vi "UDP Data Link - RTMs - Remove Channels.vi"(8 "error in (no error)":errorcluster, 11 "Node Ptr":u64 format="%.0x") -> (0 "error out":errorcluster)   [LabVIEW 2012, in "UDP Data Link System Explorer.lvlib"]
uses:
  UDP Data Link System Explorer.lvlib
  <vilib>/NI Veristand/Custom Device API/Get Item Property (I32 Array).vi
  <vilib>/NI Veristand/Custom Device API/Get Item Property (String Array).vi
  <vilib>/NI Veristand/Custom Device API/Set Item Property (I32 Array).vi
  Shared/UDP Data Link Global.vi
  <vilib>/NI Veristand/Custom Device API/Custom Device API.lvlib
  Shared/UDP Data Link Shared.lvlib
  <vilib>/NI Veristand/Custom Device Tools/Custom Device Utility Library/Custom Device Utility Library.lvlib
panel:
  in  "Tag":string
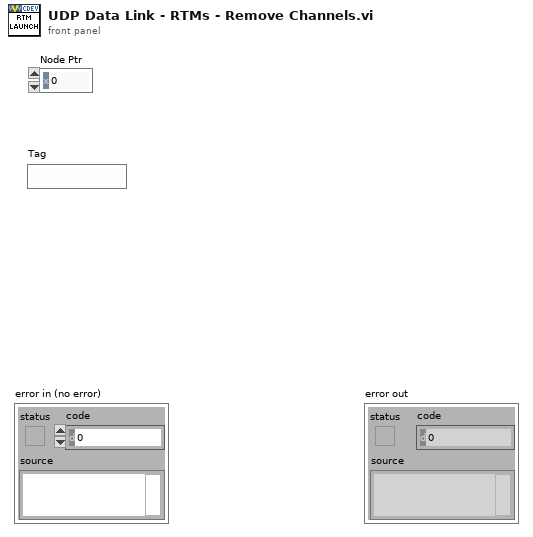
[diagram p1: front panel]
types:
  T1 = typedef "Custom Device API.lvlib/Custom Device Item Ref.ctl" = u64
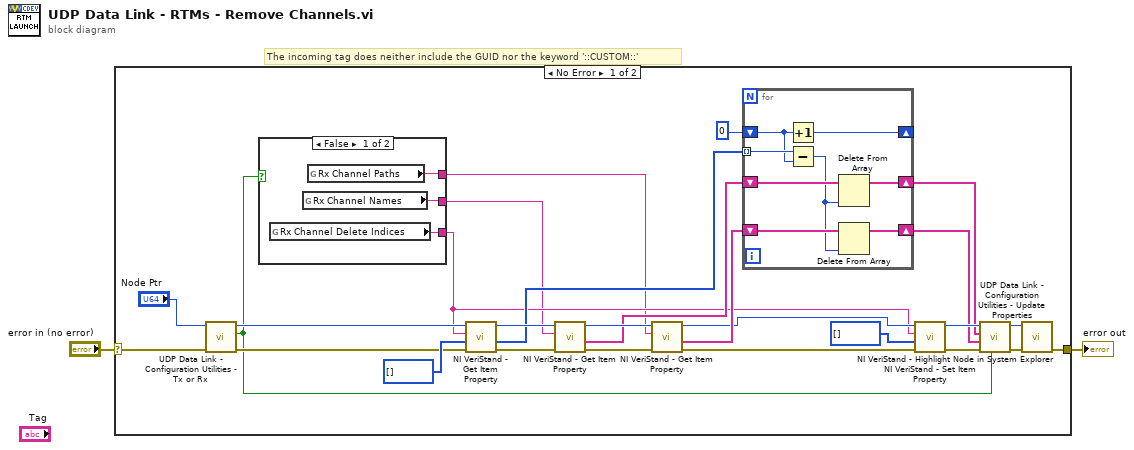
[diagram p0: block diagram]
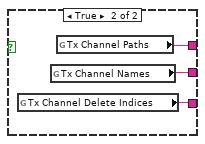
[diagram p2: hidden frame]
diagram:
  # "The incoming tag does neither include the GUID nor the keyword '::CUSTOM::'"
  n1 = case shown="No Error" "error in (no error)" {
    selector: "error in (no error)" -> [w10 w44]
    tunnel: [w18 w44] -> w2
    frame No Error {
      n2 = call "UDP Data Link - Configuration Utilities - Tx or Rx.vi"("error in (no error)"=w10, "Item Ref in"="Node Ptr") -> ("error out"=w7:errorcluster, "Tx?"=w3:bool, "Item Ref out"=w8:T1)  [unwired: 7 in]
      n3 = case shown="False" w3 {
        tunnel: [w32 w35] -> w6
        tunnel: [w31 w34] -> w5
        tunnel: [w30 w33] -> w4
        frame False {
          n4 = global read "UDP Data Link Global.vi" "Rx Channel Delete Indices"() -> (w32:string)
          n5 = global read "UDP Data Link Global.vi" "Rx Channel Names"() -> (w31:string)
          n6 = global read "UDP Data Link Global.vi" "Rx Channel Paths"() -> (w30:string)
        }
        frame True {
          n7 = global read "UDP Data Link Global.vi" "Tx Channel Delete Indices"() -> (w35:string)
          n8 = global read "UDP Data Link Global.vi" "Tx Channel Names"() -> (w34:string)
          n9 = global read "UDP Data Link Global.vi" "Tx Channel Paths"() -> (w33:string)
        }
      }
      n10 = call-poly <vilib>:"NI VeriStand - Get Item Property.vi"("error in (no error)"=w7, "Default Value"=i32[] [], "Property Name"=w6, "Item Ref in"=w8) -> ("error out"=w27:errorcluster, "Value"=w22:i32[], "Item Ref out"=w28:T1)  [unwired: 4 in, 1 out]
      n11 = call-poly <vilib>:"NI VeriStand - Get Item Property.vi"("error in (no error)"=w27, "Property Name"=w5, "Item Ref in"=w28) -> ("error out"=w26:errorcluster, "Value"=w24:string[], "Item Ref out"=w25:T1)  [unwired: 5 in, 1 out]
      n12 = call-poly <vilib>:"NI VeriStand - Get Item Property.vi"("error in (no error)"=w26, "Property Name"=w4, "Item Ref in"=w25) -> ("error out"=w21:errorcluster, "Value"=w23:string[], "Item Ref out"=w20:T1)  [unwired: 5 in, 1 out]
      n13 = for {
        shift-right: [w42] -> w12
        shift-left: w24 -> [w43]
        shift-right: [w40] -> w11
        shift-left: w23 -> [w41]
        tunnel: w22 -> [w37] mode=indexing
        shift-right: [w38] -> _
        shift-left: 0 -> [w36]
        n14 = Increment(x=w36) -> (x+1=w38:i32)
        n15 = Subtract(x=w37, y=w36) -> (x-y=w39:i32)
        n16 = Delete From Array(array=w43, index=w39) -> (array with subset deleted=w42:string[])  [unwired: 1 in, 1 out]
        n17 = Delete From Array(array=w41, index=w39) -> (array with subset deleted=w40:string[])  [unwired: 1 in, 1 out]
      }
      n18 = call-poly <vilib>:"NI VeriStand - Set Item Property.vi"("error in (no error)"=w21, "Value"=i32[] [], "Property Name"=w6, "Item Ref in"=w20) -> ("error out"=w15:errorcluster, "Item Ref out"=w13:T1)  [unwired: 5 in, 1 out]
      n19 = call "UDP Data Link - Configuration Utilities - Update Properties.vi"("Tx?"=w3, "error in (no error)"=w15, "Channel Paths"=w11, "Channel Names"=w12, "Item Ref in"=w13) -> ("error out"=w16:errorcluster, "Item Ref out"=w14:T1)  [unwired: 5 in]
      n20 = call <vilib>:"NI VeriStand - Highlight Node in System Explorer.vi"("error in (no error)"=w16, "Item Ref in"=w14) -> ("error out"=w18:errorcluster)  [unwired: 8 in, 1 out]
    }
    frame Error {
    }
  }
  "error out" <- w2
